vi "Parse All Notes.vi"(8 "error in (no error)":errorcluster, 10 "SR Cluster in":T1 {"Creation Date" format="%<%x>T"; "Last Updated" format="%<%x>T"}, 11 "result string":string) -> (0 "error out":errorcluster, 2 "SR Cluster out":T1 {"Creation Date" format="%<%x>T"; "Last Updated" format="%<%x>T"}, 3 "SR Notes array":T3[](array[typedef]) {"Note Date" format="%<%x >T"})   [LabVIEW 2018]
uses:
  Type Defs/SR Note Cluster.ctl
  Type Defs/SR Cluster.ctl
  Type Defs/SR Status.ctl
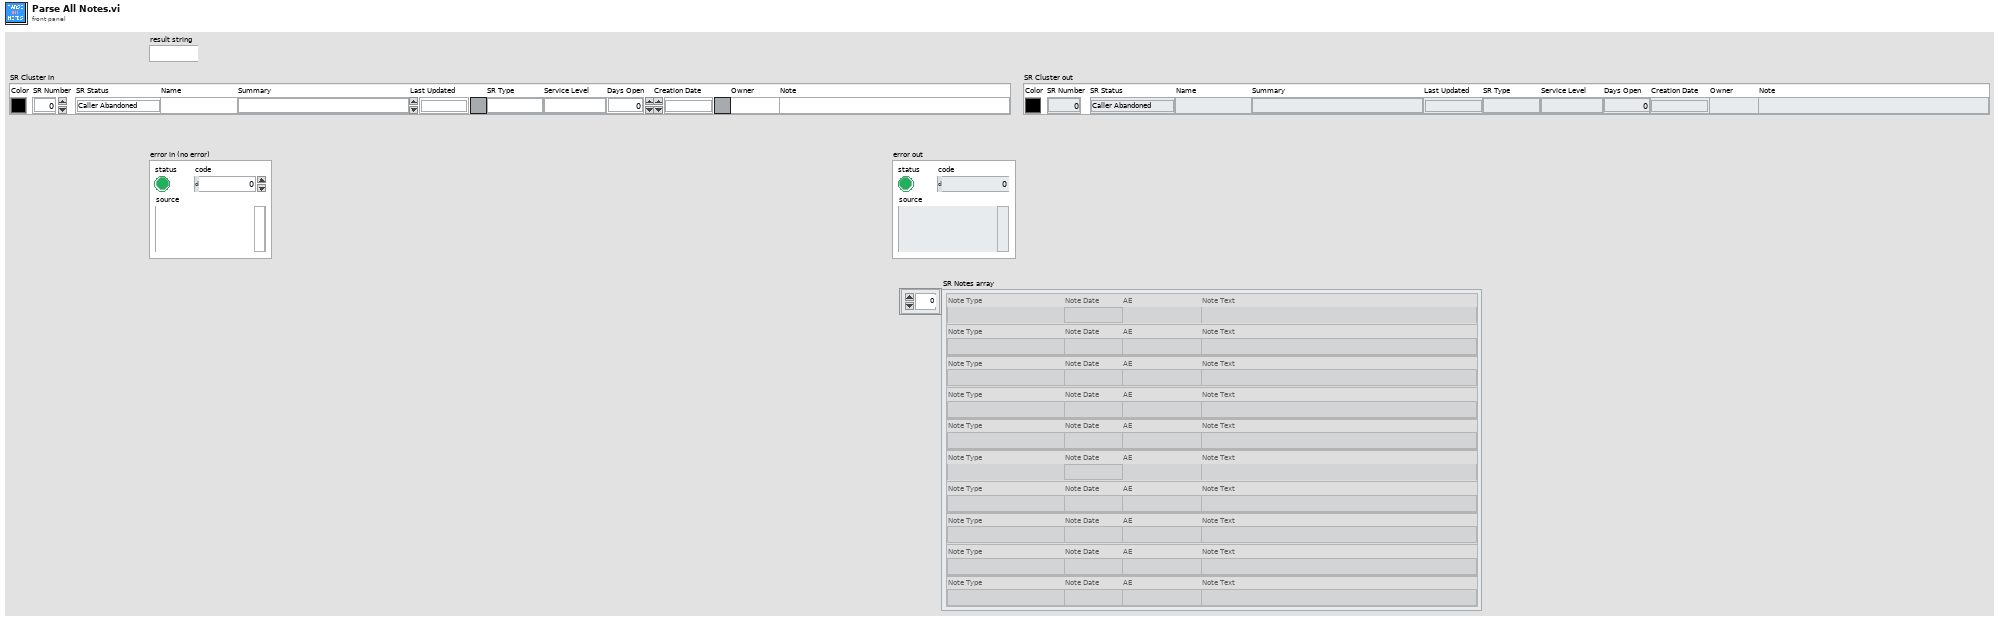
[diagram p1: front panel]
types:
  T1 = typedef "SR Cluster.ctl" = cluster{"Color":u32, "SR Number":i32, "SR Status":T2, "Name":string, "Summary":string, "Last Updated":timestamp, "SR Type":string, "Service Level":string, "Days Open":dbl, "Creation Date":timestamp, "Owner":string, "Note":string}
  T2 = typedef "SR Status.ctl" = enum16{"Caller Abandoned", "Created in Error", "Expired", "Forum Resolved AE", "Forum Resolved Customer", "IN WORK", "IN WORK Collab with AES", "IN WORK Collab with PSE", "IN WORK Collab with SE", "IN WORK Customer Added Note", "IN WORK Escalation", "IN WORK Wait on Customer", "Open", "Potentially Resolved", "Presumed Resolved", "RMA Approved for Return", "RMA Closed", "RMA Closed - DOA", "RMA In Progress", "RMA Open", "RMA Waiting on Customer", "Resolved", "Passed Off"}
  T3 = typedef "SR Note Cluster.ctl" = cluster{"Note Type":string, "Note Date":timestamp, "AE":string, "Note Text":string}
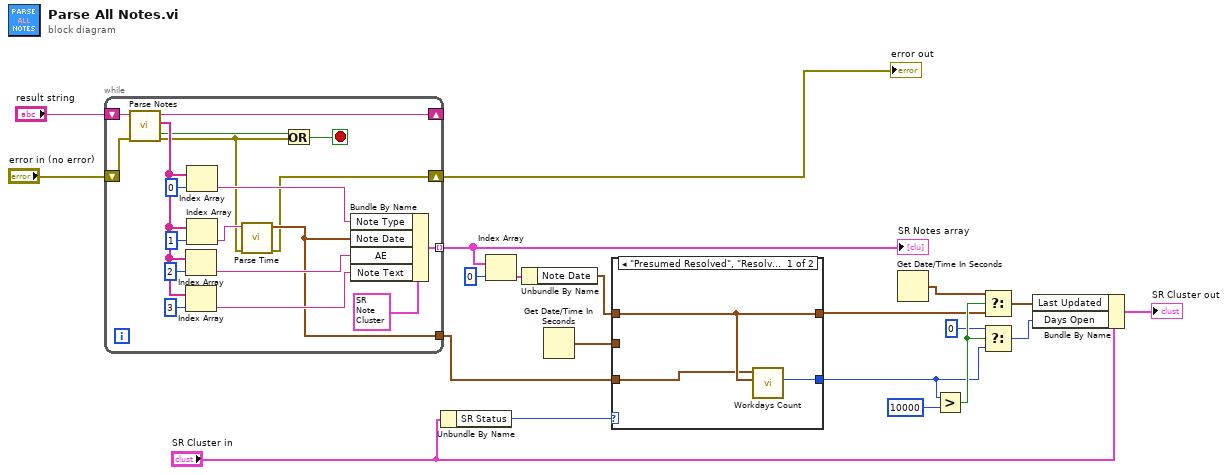
[diagram p0: block diagram]
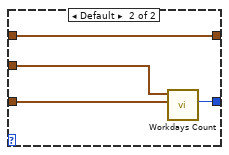
[diagram p2: hidden frame]
diagram:
  n1 = while {
    shift-right: [w38] -> _
    shift-left: "result string" -> [w39]
    tunnel: [w27] -> w14 mode=indexing
    tunnel: [w23] -> w12
    shift-right: [w22] -> w19
    shift-left: "error in (no error)" -> [w37]
    stop <- w26 stop-if-true
    n2 = call "Parse Notes.vi"("error in"=w37, "string in"=w39) -> ("error out"=w21:errorcluster, "Done Reading?"=w25:bool, "sr note out"=w36:string[], "result string out"=w38:string)  [unwired: 6 in]
    n3 = Index Array(array=w36, index=2) -> (element=w29:string)
    n4 = Index Array(array=w36, index=3) -> (element=w30:string)
    n5 = Index Array(array=w36, index=0) -> (element=w28:string)
    n6 = Index Array(array=w36, index=1) -> (element=w24:string)
    n7 = call "Parse Time.vi"("error in (no error)"=w21, "data"=w24) -> ("error out"=w22:errorcluster, "Time Stamp"=w23:timestamp)  [unwired: 8 in]
    n8 = Or(x=w25, y=w21) -> (x .or. y?=w26:bool)
    n9 = Bundle By Name(cluster=T3 {"Note Type"="", "Note Date"=timestamp(0 s since 1904-01-01), "AE"="", "Note Text"=""} ("SR Note Cluster"), "Note Type"=w28, "Note Date"=w23, "AE"=w29, "Note Text"=w30) -> (w27:T3)
  }
  "error out" <- w19
  "SR Notes array" <- w14
  n10 = Unbundle By Name("SR Cluster in") -> ("SR Status"=w13:T2)
  n11 = Index Array(array=w14, index=0) -> (element=w16:T3)
  n12 = Unbundle By Name(w16) -> ("Note Date"=w17:timestamp)
  n13 = Get Date/Time In Seconds() -> (seconds since 1Jan1904=w11:timestamp)
  n14 = case shown="\"Presumed Resolved\", \"Resolved\"" w13 {
    tunnel: w17 -> [w41 w46]
    tunnel: w12 -> [w40 w44]
    tunnel: w11 -> [_ w43]
    tunnel: [w42 w45] -> w3
    tunnel: [w41 w46] -> w5
    frame "Presumed Resolved", "Resolved" {
      n15 = call "Workdays Count.vi"("Since"=w41, "To"=w40) -> ("work days"=w42:i32)  [unwired: 8 in, 1 out]
    }
    frame Default {
      n16 = call "Workdays Count.vi"("Since"=w44, "To"=w43) -> ("work days"=w45:i32)  [unwired: 8 in, 1 out]
    }
  }
  n17 = Get Date/Time In Seconds() -> (seconds since 1Jan1904=w4:timestamp)
  n18 = Greater?(x=w3, y=10000) -> (0:w7:bool)
  n19 = Select(t=w4, s=w7, f=w5) -> (s? t:f=w6:timestamp)
  n20 = Select(t=0, s=w7, f=w3) -> (s? t:f=w8:i32)
  n21 = Bundle By Name(cluster="SR Cluster in", "Last Updated"=w6, "Days Open"=w8) -> (→"SR Cluster out":T1)
